vi "BlenderMain.vi"(8 "Error In":errorcluster, 9 "Reverse":bool, 10 "Forward":bool, 11 "Control Mode":enum16{"Open", "Control"}(ring)) -> (0 "Error Out":errorcluster)   [LabVIEW 2016]
uses:
  <vilib>/Rock Robotics/SystemInterfaces/DIO/FPGA_DIORelayChannel.ctl
  <vilib>/Rock Robotics/WPI/Relay/WPI_RelayDirection.ctl
  <vilib>/Rock Robotics/WPI/Relay/WPI_RelayValue.ctl
panel:
  # "Agitator Control Main VI\nFRC Team 34"
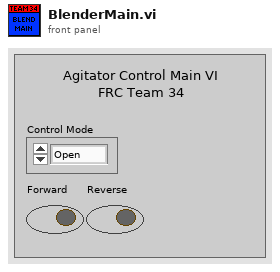
[diagram p1: front panel]
types:
  T1 = typedef "WPI_RelayDirection.ctl" = enum16{"Both directions", "Forward only", "Reverse only"}
  T2 = typedef "FPGA_DIORelayChannel.ctl" = enum8{"Relay 0", "Relay 1", "Relay 2", "Relay 3", "Invalid"}
  T3 = typedef "WPI_RelayValue.ctl" = enum16{"Off", "On", "Forward", "Reverse"}
  T4 = typedef "WPI_RelayDevRef.ctl" = cluster{"DevStatus":errorcluster, "Relay Channel":T2, "Relay Direction":T1}
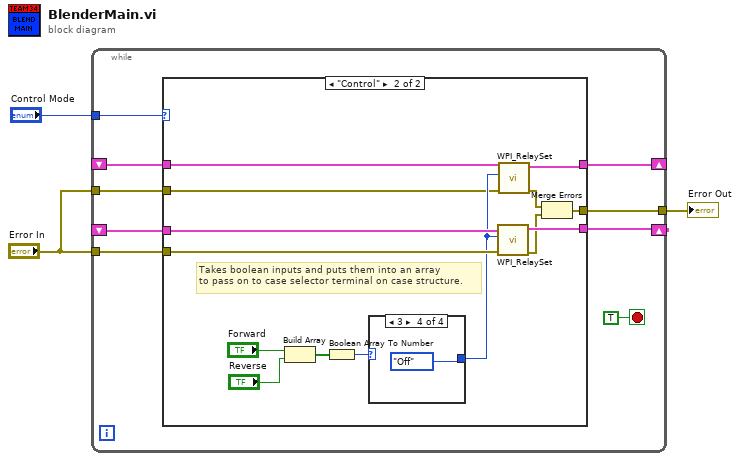
[diagram p0: block diagram]
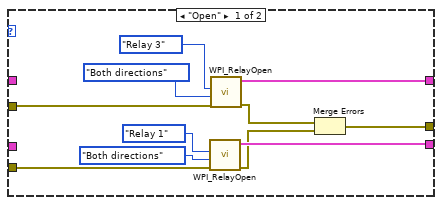
[diagram p2: hidden frame]
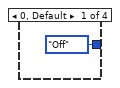
[diagram p3: hidden frame]
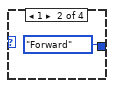
[diagram p4: hidden frame]
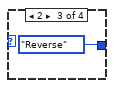
[diagram p5: hidden frame]
diagram:
  n1 = while {
    tunnel: "Control Mode" -> [w11]
    tunnel: "Error In" -> [w10]
    shift-right: [w9] -> _
    shift-left: _ -> [w8]
    shift-right: [w7] -> _
    shift-left: _ -> [w6]
    tunnel: "Error In" -> [w5]
    tunnel: [w4] -> w1
    stop <- TRUE stop-if-true
    n2 = case shown="\"Control\"" w11 {
      tunnel: w10 -> [w23 w31]
      tunnel: [w21 w32] -> w9
      tunnel: w8 -> [_ w33]
      tunnel: [w17 w28] -> w7
      tunnel: w6 -> [_ w30]
      tunnel: w5 -> [w16 w27]
      tunnel: [w13 w24] -> w4
      frame "Open" {
        n3 = call <vilib>:"WPI_RelayOpen.vi"("error in (no error)"=w23, "Relay Direction"=WPI_RelayDirection."Both directions", "Relay Channel"=FPGA_DIORelayChannel."Relay 1") -> ("error out"=w14:errorcluster, "RelayDevRef"=w21:T4)  [unwired: 7 in]
        n4 = call <vilib>:"WPI_RelayOpen.vi"("error in (no error)"=w16, "Relay Direction"=WPI_RelayDirection."Both directions", "Relay Channel"=FPGA_DIORelayChannel."Relay 3") -> ("error out"=w15:errorcluster, "RelayDevRef"=w17:T4)  [unwired: 7 in]
        n5 = Merge Errors(w15, w14) -> (w13:errorcluster)
      }
      frame "Control" {
        # "Takes boolean inputs and puts them into an array\nto pass on to case selector terminal on case structure."
        n6 = Build Array("Forward", "Reverse") -> (w35:bool[])
        n7 = Boolean Array To Number(Boolean array=w35) -> (number=w34:u32)
        n8 = case shown="3" w34 {
          tunnel: [WPI_RelayValue."Off" ("RelayValue") WPI_RelayValue."Forward" ("RelayValue") WPI_RelayValue."Reverse" ("RelayValue") WPI_RelayValue."Off" ("RelayValue")] -> w29
          frame 0, Default {
          }
          frame 1 {
          }
          frame 2 {
          }
          frame 3 {
          }
        }
        n9 = call <vilib>:"WPI_RelaySet.vi"("error in (no error)"=w31, "RelayValue"=w29, "RelayDevRef"=w33) -> ("error out"=w26:errorcluster, "RelayDevRef"=w32:T4)  [unwired: 7 in]
        n10 = call <vilib>:"WPI_RelaySet.vi"("error in (no error)"=w27, "RelayValue"=w29, "RelayDevRef"=w30) -> ("error out"=w25:errorcluster, "RelayDevRef"=w28:T4)  [unwired: 7 in]
        n11 = Merge Errors(w25, w26) -> (w24:errorcluster)
      }
    }
  }
  "Error Out" <- w1
